vi "hw4-1 topVI.vi"() -> ()   [LabVIEW 2014]
uses:
  <vilib>/Utility/miscctls.llb/LVPositionTypeDef.ctl
panel:
  out "h":dbl
  out "floor(x): largest int <= x 2":dbl
  out "Position":T1={"Left"=452, "Top"=-38}
  out "t":dbl
  out "k":dbl
  out "h":dbl
  out "a":dbl
  out "position":cluster{i32, dbl}
  out "floor(x): largest int <= x":dbl
  out "x2":dbl
  out "y3":dbl
  out "x3":dbl
  in  "percentage threshold \nof energy remained":dbl=40.0
  in  "percentage of\nenergy loss":dbl=30.0
  in  "initial angle\n(degree)":dbl=30.0
  in  "initial velocity\n(m/s)":dbl=45.0
  out "CannonBall":bool=TRUE
  # "Assume the canninball mass = 1 kg"
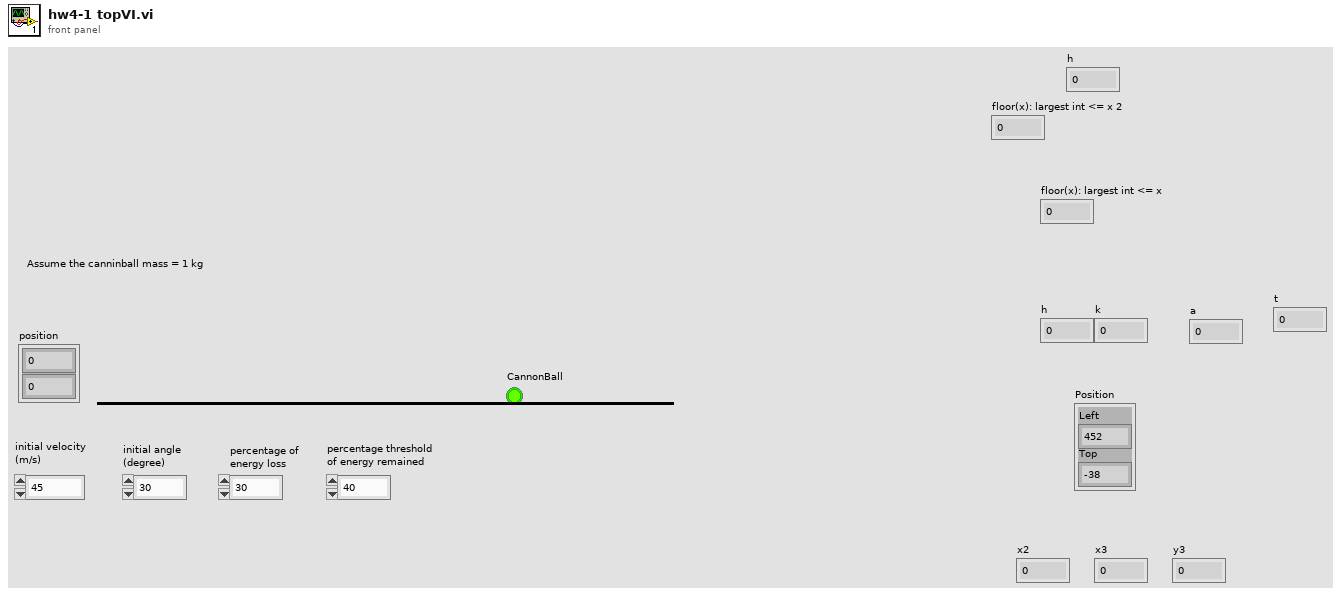
[diagram p1: front panel]
types:
  T1 = typedef "LVPositionTypeDef.ctl" = cluster{"Left":i32, "Top":i32}
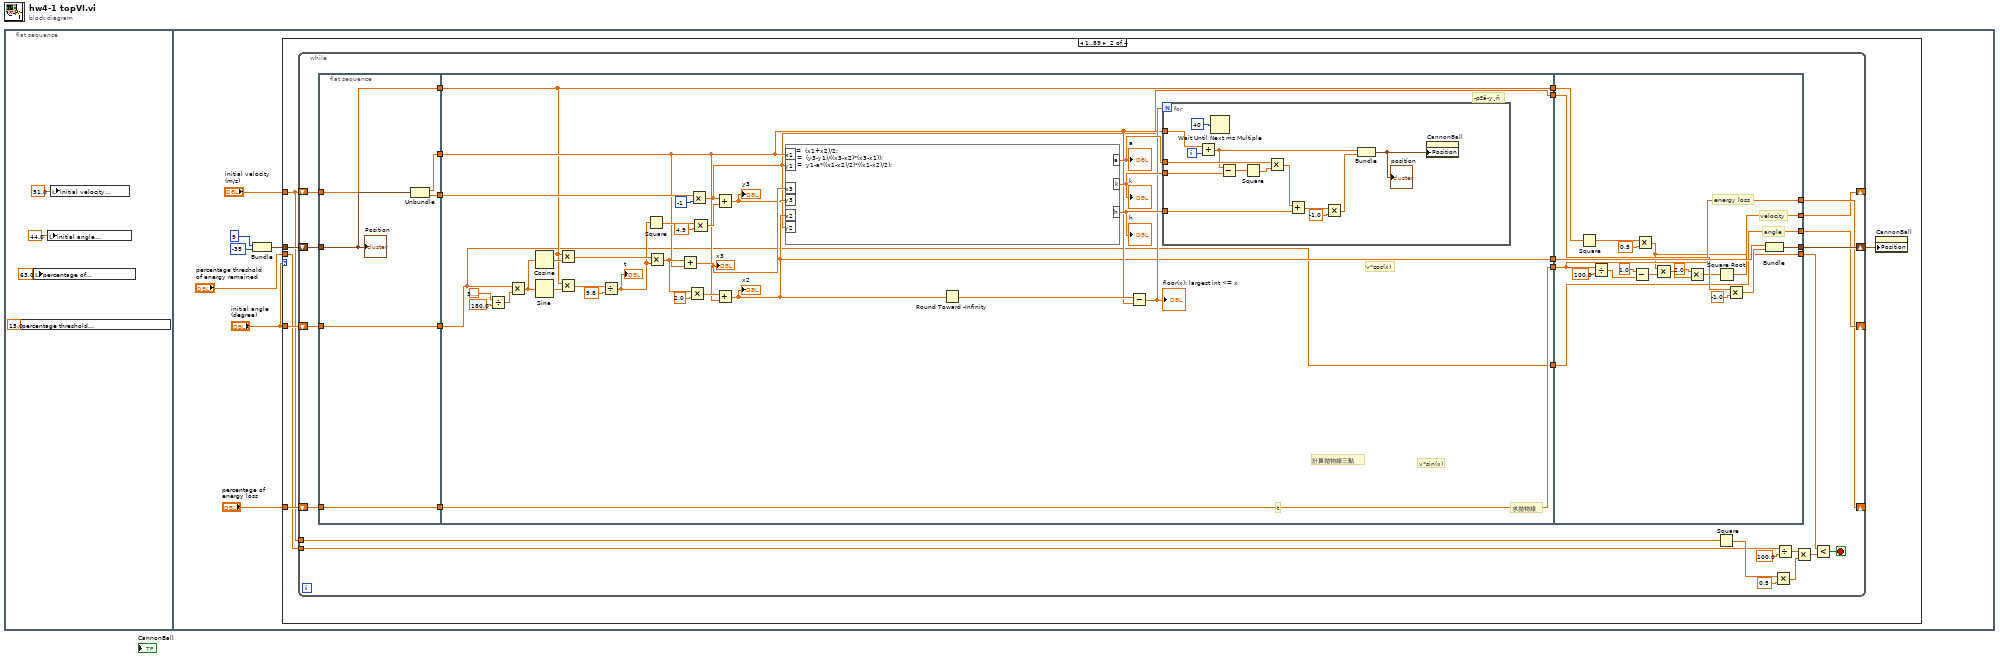
[diagram p0: block diagram]
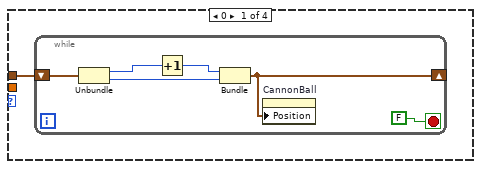
[diagram p2: hidden frame]
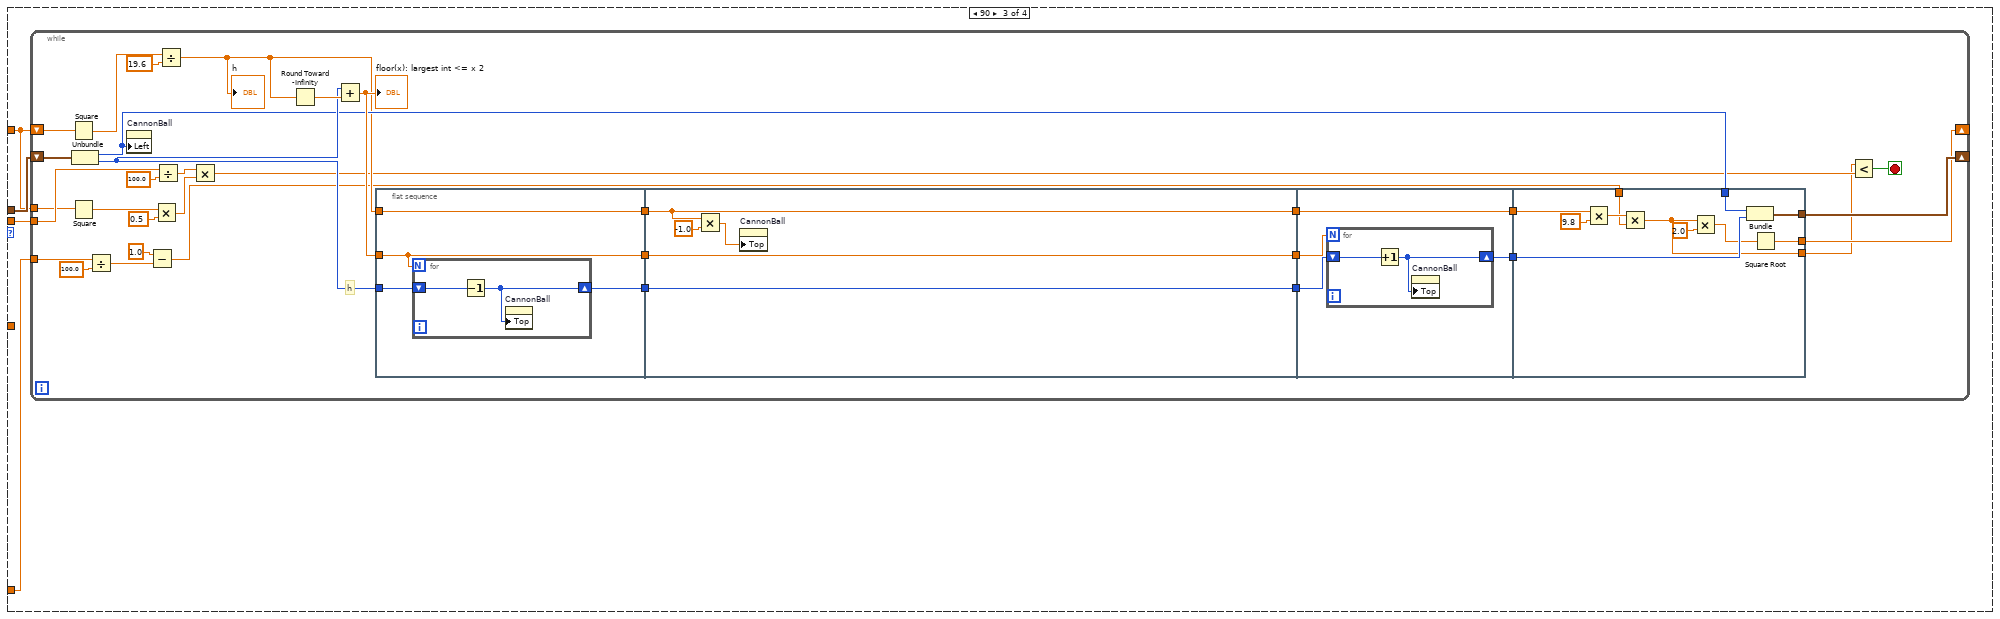
[diagram p3: hidden frame]
diagram:
  n1 = flat-sequence {
    frame #0 {
      n2 = local write "percentage threshold \nof energy remained"(15.0 ("percentage threshold \nof energy remained")) -> ()
      n3 = local write "percentage of\nenergy loss"(63.0 ("percentage of\nenergy loss")) -> ()
      n4 = local write "initial angle\n(degree)"(44.0 ("initial angle\n(degree)")) -> ()
      n5 = local write "initial velocity\n(m/s)"(51.0 ("initial velocity\n(m/s)")) -> ()
    }
    frame #1 {
      n6 = Bundle(9, -35) -> (w7:cluster{i32, i32})  [unwired: 1 in]
      n7 = case shown="1..89" "initial angle\n(degree)" {
        tunnel: "percentage of\nenergy loss" -> [_ w23 w125 _]
        tunnel: "initial velocity\n(m/s)" -> [_ w20 w123 _]
        tunnel: w7 -> [w12 w22 w126 _]
        tunnel: "initial angle\n(degree)" -> [_ w21 _ _]
        tunnel: "percentage threshold \nof energy remained" -> [_ w19 w124 _]
        frame 0 {
          n8 = while {
            shift-right: [w13] -> _
            shift-left: w12 -> [w17]
            stop <- FALSE stop-if-true
            n9 = Unbundle(w17) -> (w18:i32, w15:i32)
            n10 = Increment(x=w18) -> (x+1=w16:i32)
            n11 = Bundle(w16, w15) -> (w13:cluster{i32, i32})  [unwired: 1 in]
            n12 = property on="CannonBall" class="Bool (strict)"("Position"=w13) -> ()  [unwired: 2 in, 2 out]
          }
        }
        frame 1..89 {
          n13 = while {
            shift-right: [w42] -> w24
            shift-left: w22 -> [w41]
            shift-right: [w40] -> _
            shift-left: w21 -> [w39]
            shift-right: [w38] -> _
            shift-left: w23 -> [w37]
            shift-right: [w36] -> _
            shift-left: w20 -> [w35]
            tunnel: w20 -> [w31]
            tunnel: w19 -> [w25]
            stop <- w32 stop-if-true
            n14 = flat-sequence {
              tunnel: [w58] -> w52
              tunnel: [w57] -> w51
              tunnel: w41 -> [w56]
              tunnel: w39 -> [w55]
              tunnel: [w55] -> w50
              tunnel: w35 -> [w54]
              tunnel: [w54] -> w49
              tunnel: w37 -> [w53]
              tunnel: [w53] -> w48
              tunnel: w52 -> [w64]
              tunnel: w51 -> [w68]
              tunnel: [w63] -> w47
              tunnel: [w62] -> w46
              tunnel: w50 -> [w59]
              tunnel: w49 -> [w60]
              tunnel: w48 -> [w61]
              tunnel: [w61] -> w45
              tunnel: [w60] -> w44
              tunnel: [w59] -> w43
              tunnel: w47 -> [w122]
              tunnel: w46 -> [w120]
              tunnel: w45 -> [w109]
              tunnel: [w118] -> w42
              tunnel: w44 -> [w116]
              tunnel: [w111] -> w36
              tunnel: [w109] -> w38
              tunnel: [w110] -> w40
              tunnel: w43 -> [w110]
              tunnel: [w104] -> w33
              frame #0 {
                n15 = Unbundle(w56) -> (w58:dbl, w57:dbl)
                "Position" <- w56
              }
              frame #1 {
                # "­pºâ­y¸ñ"
                # "求拋物線"
                # "計算拋物線三點"
                # "t"
                # "v*cos(x)"
                # "v*sin(x)"
                n16 = Divide(x=3.141592653589793, y=180.0) -> (x/y=w87:dbl)
                n17 = Multiply(x=w59, y=w87) -> (x*y=w86:dbl)
                n18 = Cosine(x=w86) -> (cos(x)=w84:dbl)
                n19 = Sine(x=w86) -> (sin(x)=w85:dbl)
                n20 = Multiply(x=w60, y=w84) -> (x*y=w82:dbl)
                n21 = Multiply(x=w60, y=w85) -> (x*y=w81:dbl)
                n22 = Divide(x=w81, y=9.8) -> (x/y=w73:dbl)
                "t" <- w73
                n23 = Square(x=w73) -> (x^2=w72:dbl)
                n24 = Multiply(x=w82, y=w73) -> (x*y=w79:dbl)
                n25 = Add(x=w79, y=w64) -> (x+y=w77:dbl)
                "x3" <- w77
                n26 = Multiply(x=w79, y=2.0) -> (x*y=w78:dbl)
                n27 = Multiply(x=w68, y=-1) -> (x*y=w62:dbl)
                n28 = Multiply(x=w72, y=4.9) -> (x*y=w70:dbl)
                n29 = Add(x=w62, y=w70) -> (x+y=w69:dbl)
                "y3" <- w69
                n30 = Add(x=w78, y=w64) -> (x+y=w63:dbl)
                "x2" <- w63
                n31 = formula code="k =  (x1+x2)/2;\na =  (y3-y1)/((x3-x2)*(x3-x1));\nh =  y1-a*((x1-x2)/2)*((x1-x2)/2);"("x1"=w64, "y1"=w62, "x3"=w77, "y3"=w69, "x2"=w63, "y2"=w62) -> ("a"=w76:dbl, "k"=w75:dbl, "h"=w74:dbl)
                "a" <- w76
                "h" <- w74
                "k" <- w75
                n32 = Round Toward -Infinity(1:w63) -> (0:w66:dbl)
                n33 = Subtract(x=w66, y=w64) -> (x-y=w65:dbl)
                "floor(x): largest int <= x" <- w65
                n34 = for {
                  N: w65 -> [_]
                  tunnel: w76 -> [w98]
                  tunnel: w75 -> [w101]
                  tunnel: w74 -> [w97]
                  tunnel: w64 -> [w90]
                  i -> [w92]
                  n35 = Add(x=w90, y=w92) -> (x+y=w91:dbl)
                  n36 = Wait Until Next ms Multiple(millisecond multiple=u32 40) -> ()  [unwired: 1 out]
                  n37 = Subtract(x=w91, y=w101) -> (x-y=w100:dbl)
                  n38 = Square(x=w100) -> (x^2=w99:dbl)
                  n39 = Multiply(x=w98, y=w99) -> (x*y=w96:dbl)
                  n40 = Add(x=w96, y=w97) -> (x+y=w94:dbl)
                  n41 = Multiply(x=w94, y=-1.0) -> (x*y=w93:dbl)
                  n42 = Bundle(w91, w93) -> (w103:cluster{dbl, dbl})  [unwired: 1 in]
                  "position" <- w103
                  n43 = property on="CannonBall" class="Bool (strict)"("Position"=w103) -> ()  [unwired: 2 in, 2 out]
                }
              }
              frame #2 {
                # "angle"
                # "energy loss"
                # "velocity"
                n44 = Square(x=w116) -> (x^2=w115:dbl)
                n45 = Divide(x=w109, y=100.0) -> (x/y=w107:dbl)
                n46 = Subtract(x=1.0, y=w107) -> (x-y=w105:dbl)
                n47 = Multiply(x=w115, y=0.5) -> (x*y=w104:dbl)
                n48 = Multiply(x=w104, y=w105) -> (x*y=w114:dbl)
                n49 = Multiply(x=2.0, y=w114) -> (x*y=w112:dbl)
                n50 = Square Root(x=w112) -> (sqrt(x)=w111:dbl)
                n51 = Multiply(x=w120, y=-1.0) -> (x*y=w119:dbl)
                n52 = Bundle(w122, w119) -> (w118:cluster{dbl, dbl})  [unwired: 1 in]
              }
            }
            n53 = Square(x=w31) -> (x^2=w30:dbl)
            n54 = Multiply(x=w30, y=0.5) -> (x*y=w28:dbl)
            n55 = Divide(x=w25, y=100.0) -> (x/y=w27:dbl)
            n56 = Multiply(x=w27, y=w28) -> (x*y=w34:dbl)
            n57 = Less?(x=w33, y=w34) -> (x < y?=w32:bool)
          }
          n58 = property on="CannonBall" class="Bool (strict)"("Position"=w24) -> ()  [unwired: 2 in, 2 out]
        }
        frame 90 {
          n59 = while {
            shift-right: [w137] -> _
            shift-left: w123 -> [w150]
            shift-right: [w146] -> _
            shift-left: w126 -> [w149]
            tunnel: w125 -> [w139]
            tunnel: w124 -> [w129]
            tunnel: w123 -> [w128]
            stop <- w127 stop-if-true
            # "h"
            n60 = Square(x=w150) -> (x^2=w155:dbl)
            n61 = Square(x=w128) -> (x^2=w135:dbl)
            n62 = Unbundle(w149) -> (w147:i32, w152:i32)
            n63 = Divide(x=w139, y=100.0) -> (x/y=w141:dbl)
            n64 = property on="CannonBall" class="Bool (strict)"("Left"=w147) -> ()  [unwired: 2 in, 2 out]
            n65 = Subtract(x=1.0, y=w141) -> (x-y=w138:dbl)
            n66 = Multiply(x=w135, y=0.5) -> (x*y=w133:dbl)
            n67 = Divide(x=w129, y=100.0) -> (x/y=w132:dbl)
            n68 = Divide(x=w155, y=19.6) -> (x/y=w143:dbl)
            "h" <- w143
            n69 = Multiply(x=w132, y=w133) -> (x*y=w136:dbl)
            n70 = Round Toward -Infinity(1:w143) -> (0:w153:dbl)
            n71 = Add(x=w152, y=w153) -> (x+y=w151:dbl)
            "floor(x): largest int <= x 2" <- w151
            n72 = flat-sequence {
              tunnel: w152 -> [w162]
              tunnel: w151 -> [w163]
              tunnel: w143 -> [w164]
              tunnel: [w164] -> w160
              tunnel: [w163] -> w159
              tunnel: [w161] -> w158
              tunnel: w160 -> [w167]
              tunnel: [w169] -> w157
              tunnel: w159 -> [w169]
              tunnel: [w168] -> w156
              tunnel: w158 -> [w168]
              tunnel: [w167] -> w145
              tunnel: w157 -> [w175]
              tunnel: w156 -> [w174]
              tunnel: [w173] -> w148
              tunnel: w145 -> [w172]
              tunnel: [w172] -> w144
              tunnel: w148 -> [w188]
              tunnel: w147 -> [w187]
              tunnel: [w186] -> w146
              tunnel: w144 -> [w185]
              tunnel: w138 -> [w182]
              tunnel: [w179] -> w137
              tunnel: [w178] -> w130
              frame #0 {
                n73 = for {
                  N: w163 -> [_]
                  shift-right: [w165] -> w161
                  shift-left: w162 -> [w166]
                  n74 = Decrement(x=w166) -> (x-1=w165:i32)
                  n75 = property on="CannonBall" class="Bool (strict)"("Top"=w165) -> ()  [unwired: 2 in, 2 out]
                }
              }
              frame #1 {
                n76 = Multiply(x=w167, y=-1.0) -> (x*y=w171:dbl)
                n77 = property on="CannonBall" class="Bool (strict)"("Top"=w171) -> ()  [unwired: 2 in, 2 out]
              }
              frame #2 {
                n78 = for {
                  N: w175 -> [_]
                  shift-right: [w176] -> w173
                  shift-left: w174 -> [w177]
                  n79 = Increment(x=w177) -> (x+1=w176:i32)
                  n80 = property on="CannonBall" class="Bool (strict)"("Top"=w176) -> ()  [unwired: 2 in, 2 out]
                }
              }
              frame #3 {
                n81 = Multiply(x=w185, y=9.8) -> (x*y=w183:dbl)
                n82 = Multiply(x=w183, y=w182) -> (x*y=w178:dbl)
                n83 = Multiply(x=w178, y=2.0) -> (x*y=w180:dbl)
                n84 = Bundle(w187, w188) -> (w186:cluster{i32, i32})  [unwired: 1 in]
                n85 = Square Root(x=w180) -> (sqrt(x)=w179:dbl)
              }
            }
            n86 = Less?(x=w130, y=w136) -> (x < y?=w127:bool)
          }
        }
        frame Default {
        }
      }
    }
  }
